vi "Event Init.vi"(6 "Event Self":map{string, refnum<data-value>}(c390), 8 "Queue Nested":map{string, refnum<data-value>}(c390), 9 "Queue Self":map{string, refnum<data-value>}(c390), 10 "Queue Caller":map{string, refnum<data-value>}(c390)) -> (3 "Base Event Actor out":refnum<class "Base Event Actor.lvclass">)   [LabVIEW 2021, in "jettl.lvlib" / "Base Event Actor.lvclass"]
uses:
  Base Event Actor.lvclass
  Msg/Msg/Msg.lvclass
  Event State/Nominal Event State/Nominal Event State.lvclass
  C:/git/jettl/src/jettl/Event State/Event State/Event State.lvclass
  Base Event Actor.lvclass/Base Event Actor.ctl
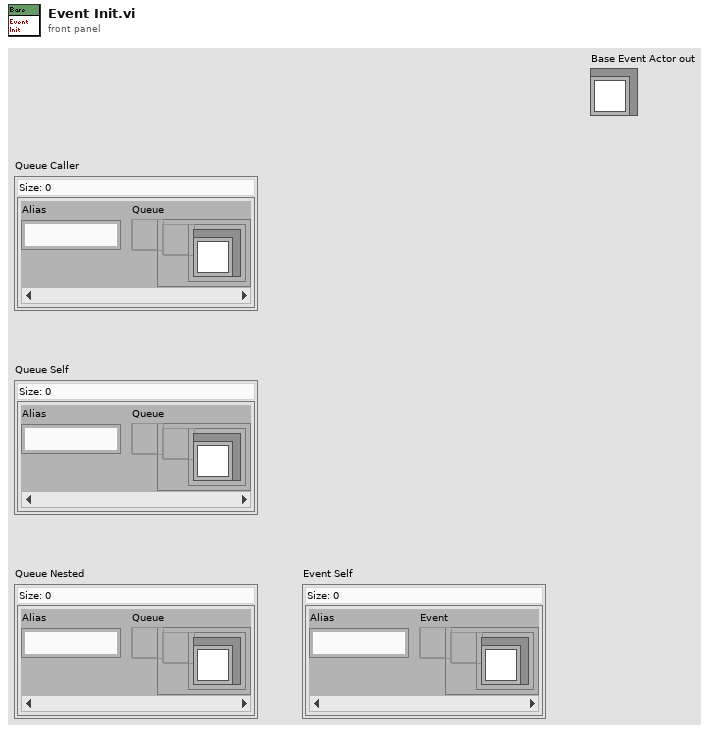
[diagram p1: front panel]
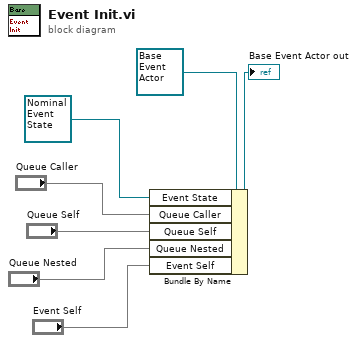
[diagram p0: block diagram]
diagram:
  n1 = Bundle By Name(cluster=refnum<class "Base Event Actor.lvclass"> refnum ("jettl Event Actor out"), "Event State"=refnum<class "Nominal Event State.lvclass"> refnum ("jettl.lvlib:Nominal Event State.lvclass"), "Queue Caller"="Queue Caller", "Queue Self"="Queue Self", "Queue Nested"="Queue Nested", "Event Self"="Event Self") -> (→"Base Event Actor out":refnum<class "Base Event Actor.lvclass">)
